vi "COMn单步调试对话框.vi"() -> ()   [LabVIEW 2016, in "斯坦道CODMn新电路板.lvlib"]
uses:
  <vilib>/Utility/miscctls.llb/LVPointTypeDef.ctl
panel:
  in  "停止":bool
  in  "CODMn调试控件V3":cluster{"数值":u16[], "模式":enum32{"测试模式", "流程模式"}}(xcontrol)
  in  "退出":bool
  in  "启动":bool
  # "CODMn单步调试界面"
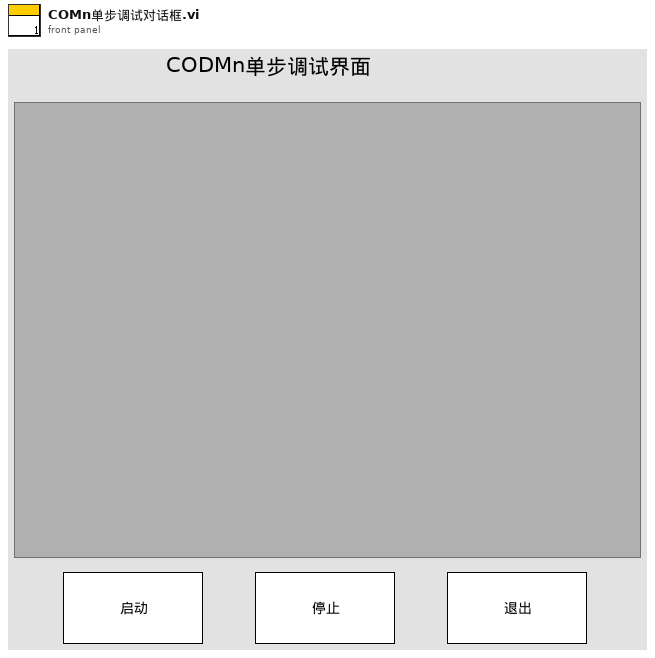
[diagram p1: front panel]
types:
  T1 = typedef "LVPointTypeDef.ctl" = cluster{"Horizontal":i16, "Vertical":i16}
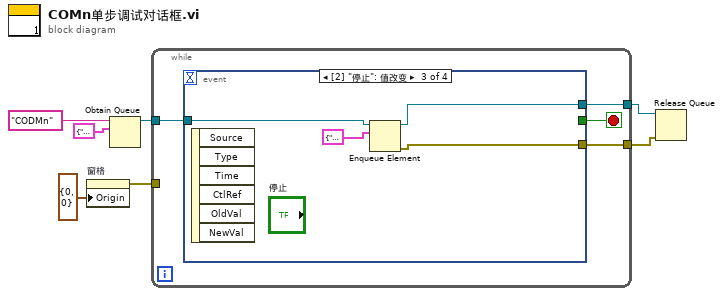
[diagram p0: block diagram]
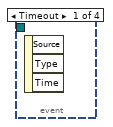
[diagram p2: hidden frame]
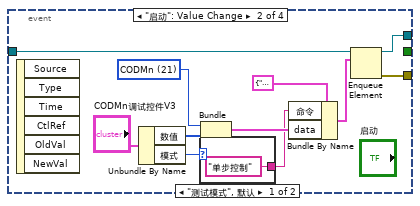
[diagram p3: hidden frame]
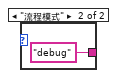
[diagram p4: hidden frame]
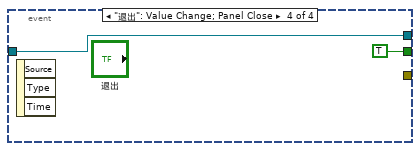
[diagram p5: hidden frame]
diagram:
  n1 = property on="窗格" class="Pane"("Origin"=T1 {"Horizontal"=0, "Vertical"=0} ("原点")) -> (error out=w2:errorcluster)  [unwired: 2 in, 1 out]
  n2 = Obtain Queue(name (unnamed)="CODMn" ("名称（未命名）"), element data type=cluster{"命令":string, "data":variant} {"命令"="", "data"=variant}) -> (queue out=w5:refnum<queue>)  [unwired: 3 in, 2 out]
  n3 = while {
    tunnel: w5 -> [w10]
    tunnel: [w9] -> w4
    tunnel: [w8] -> w3
    tunnel: w2 -> [_]
    stop <- w11 stop-if-true
    n4 = event shown="[2] \"停止\": 值改变" {
      selector: _ -> [_ _ _ _]
      dyn-events: _ -> [_ _ _ _]
      timeout: _ -> [_ _ _ _]
      tunnel: [_ _ _ TRUE] -> w11
      tunnel: w10 -> [_ w18 w27 w29]
      tunnel: [_ w17 w26 w29] -> w9
      tunnel: [_ w16 w25 _] -> w8
      event Timeout {
        n5 = event-data() -> ()  [unwired: 1 in, 3 out]
      }
      event "启动": Value Change {
        w20 = u16 21 items=["CODMn"=21, "总磷"=1, "氨氮"=3] ("站号")
        n6 = event-data() -> ()  [unwired: 1 in, 6 out]
        n7 = Unbundle By Name("CODMn调试控件V3") -> ("数值"=w15:u16[], "模式"=w13:enum32{"测试模式", "流程模式"})
        n8 = case shown="\"测试模式\", 默认" w13 {
          tunnel: ["单步控制" ("命令") "debug" ("命令")] -> w12
          frame "测试模式", Default {
          }
          frame "流程模式" {
          }
        }
        n9 = Bundle("站号"=w20, "数值"=w15) -> (w19:cluster{"站号":u16, "数值":u16[]})  [unwired: 1 in]
        n10 = Bundle By Name(cluster=cluster{"命令":string, "data":variant} {"命令"="", "data"=variant} ("元素"), "命令"=w12, "data"=w19) -> (w21:cluster{"命令":string, "data":variant})
        n11 = Enqueue Element(queue=w18, element=w21) -> (queue out=w17:refnum<queue>, error out=w16:errorcluster)  [unwired: 2 in, 1 out]
      }
      event "停止": Value Change {
        n12 = event-data() -> ()  [unwired: 1 in, 6 out]
        n13 = Enqueue Element(queue=w27, element=cluster{"命令":string, "data":variant} {"命令"="启动", "data"=variant(cluster{"站号":u16, "控制命令":u16[]} {"站号"=21, "控制命令"=[2816]})} ("启动命令")) -> (queue out=w26:refnum<queue>, error out=w25:errorcluster)  [unwired: 2 in, 1 out]
      }
      event "退出": Value Change; Panel Close {
        n14 = event-data() -> ()  [unwired: 1 in, 3 out]
      }
    }
  }
  n15 = Release Queue(queue=w4, error in (no error)=w3) -> ()  [unwired: 1 in, 3 out]
